vi "Make A selection of object.vi"(8 "error in (no error)":errorcluster, 11 "Data":T1) -> (0 "error out":errorcluster)   [LabVIEW 2014, in "SmartPalette.lvlib"]
uses:
  SmartPalette.lvlib
  Controls/Data To Predictor.ctl
  Controls/GObjectDetail.ctl
  <vilib>/Utility/traverseref.llb/TRef TravTarget.ctl
  <vilib>/regexp/Match Regular Expression.xnode
  <vilib>/Utility/traverseref.llb/VI Scripting - Traverse.lvlib
panel:
  # "ToDo:\nComplete this\n- Get the nodes with UID \n- Make the objected selected \n- Trigering the plugingnext VI will take care"
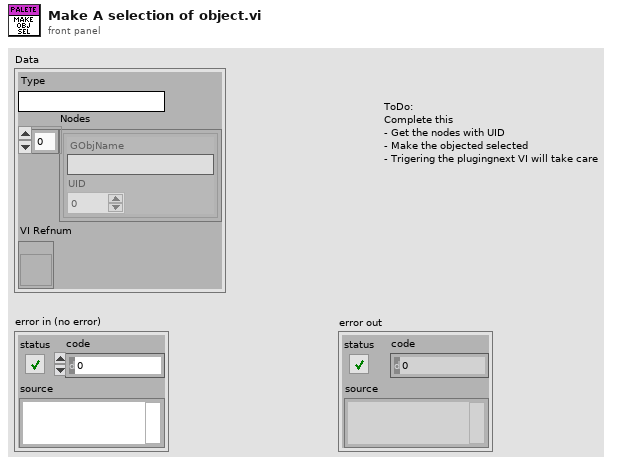
[diagram p1: front panel]
types:
  T1 = typedef "SmartPalette.lvlib/Data To Predictor.ctl" = cluster{"Type":string, "Nodes":T2[], "VI Refnum":refnum<vi>}
  T2 = typedef "SmartPalette.lvlib/GObjectDetail.ctl" = cluster{"GObjName":string, "UID":i32}
  T3 = typedef "TRef TravTarget.ctl" = enum16{"FP", "BD", "Other"}
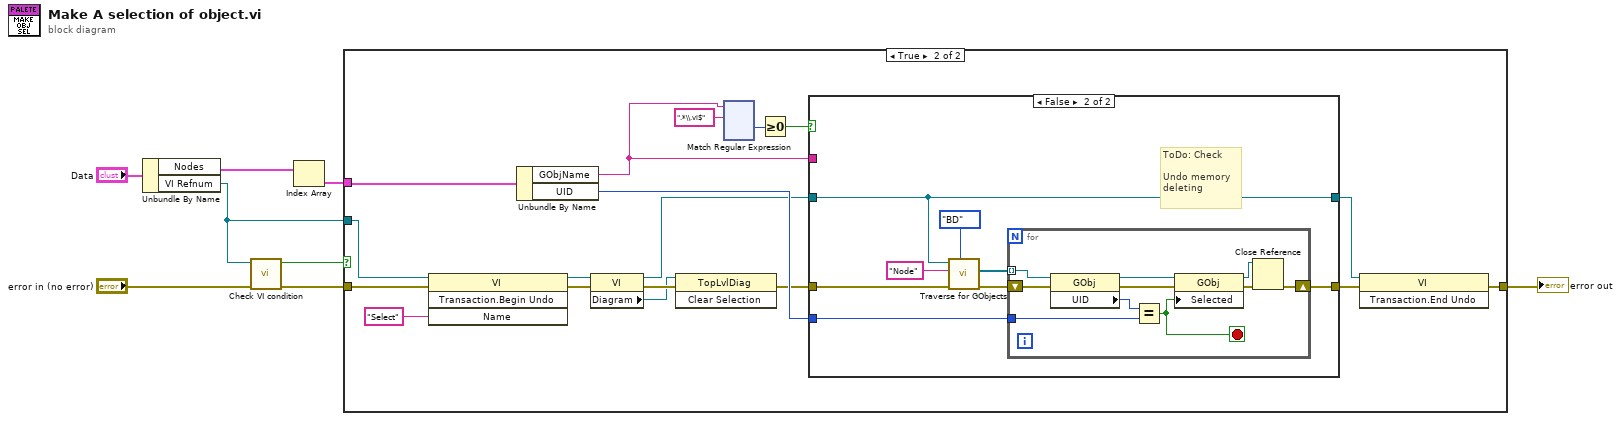
[diagram p0: block diagram]
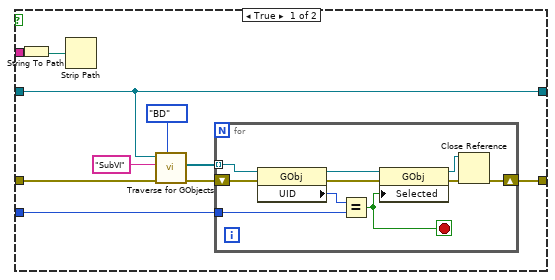
[diagram p3: hidden frame]
diagram:
  n1 = Unbundle By Name("Data") -> ("Nodes"=w2:T2[], "VI Refnum"=w4:refnum<vi>)
  n2 = call "Check VI condition.vi"("error in (no error)"="error in (no error)", "This VI"=w4) -> ("error out"=w6:errorcluster, "Good To read BD?"=w5:bool)  [unwired: 8 in]
  n3 = Index Array(array=w2) -> (element=w7:T2)  [unwired: 1 in]
  n4 = case shown="True" w5 {
    tunnel: w7 -> [_ w27]
    tunnel: [w9 w14] -> w3
    tunnel: w6 -> [w9 w13]
    tunnel: w4 -> [_ w18]
    frame False {
    }
    frame True {
      n5 = invoke class="VI" method="Transaction.Begin Undo"(reference=w18, error in=w13, "Name"="Select") -> (reference out=w11:refnum<vi>, error out=w12:errorcluster)  [unwired: 1 in, 2 out]
      n6 = Unbundle By Name(w27) -> ("GObjName"=w20:string, "UID"=w26:i32)
      n7 = property class="VI"(reference=w11, error in=w12) -> (reference out=w16:refnum<vi>, error out=w25:errorcluster, "Diagram"=w23:refnum<vi>)
      n8 = invoke class="TopLvlDiag" method="Clear Selection"(reference=w23, error in=w25) -> (error out=w24:errorcluster)  [unwired: 1 in, 2 out]
      n9 = xnode "Match Regular Expression"("input string"=w20, "regular expression"=".*\\.vi$") -> ("offset past match"=w21:i32)  [unwired: 4 in, 4 out]
      n10 = Greater Or Equal To 0?(x=w21) -> (x >= 0?=w19:bool)
      n11 = case shown="False" w19 {
        tunnel: w20 -> [w151 _]
        tunnel: w16 -> [w142 w162]
        tunnel: w24 -> [w143 w164]
        tunnel: [w146 w167] -> w15
        tunnel: w26 -> [w144 w165]
        tunnel: [w142 w162] -> w10
        frame True {
          n12 = String To Path(string=w151) -> (path=w148:path)
          n13 = Strip Path(path=w148) -> ()  [unwired: 2 out]
          n14 = call <vilib>:"Traverse for GObjects.vi"("Traverse Target"=TRef_TravTarget."BD", "error in (no error)"=w143, "Class Name"="SubVI" ("Nodes"), "VI Refnum"=w142) -> ("error out"=w149:errorcluster, "References"=w145:refnum<vi>[])  [unwired: 4 in, 2 out]
          n15 = for {
            tunnel: w145 -> [w160] mode=indexing
            shift-right: [w153] -> w146
            shift-left: w149 -> [w161]
            tunnel: w144 -> [w159]
            stop <- w154 stop-if-true
            n16 = property class="GObj"(reference=w160, error in=w161) -> (reference out=w155:refnum<vi>, error out=w157:errorcluster, "UID"=w158:i32)
            n17 = Equal?(x=w158, y=w159) -> (x = y?=w154:bool)
            n18 = property class="GObj"(reference=w155, error in=w157, "Selected"=w154) -> (reference out=w152:refnum<vi>, error out=w156:errorcluster)
            n19 = Close Reference(reference=w152, error in (no error)=w156) -> (error out=w153:errorcluster)
          }
        }
        frame False {
          # "ToDo: Check\n \nUndo memory\ndeleting"
          n20 = call <vilib>:"Traverse for GObjects.vi"("Traverse Target"=TRef_TravTarget."BD", "error in (no error)"=w164, "Class Name"="Node", "VI Refnum"=w162) -> ("error out"=w169:errorcluster, "References"=w166:refnum<vi>[])  [unwired: 4 in, 2 out]
          n21 = for {
            tunnel: w166 -> [w177] mode=indexing
            shift-right: [w171] -> w167
            shift-left: w169 -> [w179]
            tunnel: w165 -> [w176]
            stop <- w172 stop-if-true
            n22 = property class="GObj"(reference=w177, error in=w179) -> (reference out=w173:refnum<vi>, error out=w178:errorcluster, "UID"=w175:i32)
            n23 = Equal?(x=w175, y=w176) -> (x = y?=w172:bool)
            n24 = property class="GObj"(reference=w173, error in=w178, "Selected"=w172) -> (reference out=w170:refnum<vi>, error out=w174:errorcluster)
            n25 = Close Reference(reference=w170, error in (no error)=w174) -> (error out=w171:errorcluster)
          }
        }
      }
      n26 = invoke class="VI" method="Transaction.End Undo"(reference=w10, error in=w15) -> (error out=w14:errorcluster)  [unwired: 1 in, 2 out]
    }
  }
  "error out" <- w3
